vi "Write Content Bounds Width.vi"(8 "error in (no error)":errorcluster, 10 "ContentBounds.Width":u32, 11 "SceneGraphDisplay.lvclass in":refnum<class "SceneGraphDisplay.lvclass">) -> (0 "error out":errorcluster, 3 "SceneGraphDisplay.lvclass out":refnum<class "SceneGraphDisplay.lvclass">)   [LabVIEW 2015, in "SceneGraphDisplay.lvclass"]
uses:
  SceneGraphDisplay.lvclass
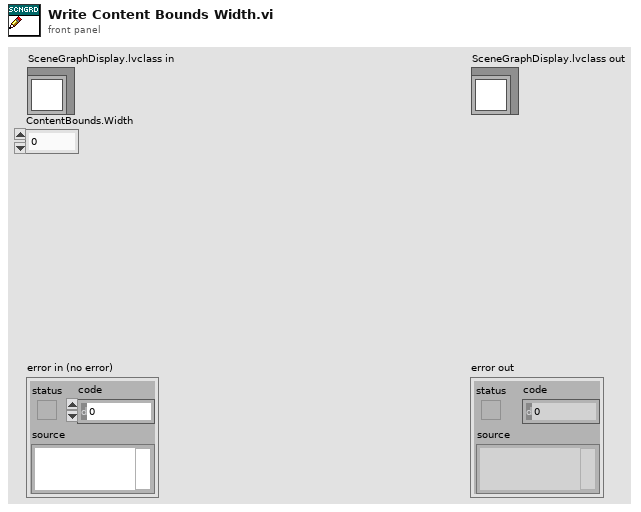
[diagram p1: front panel]
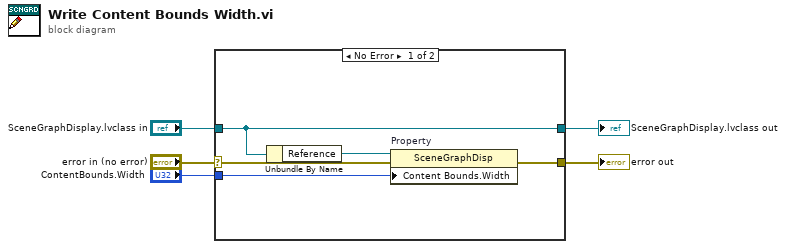
[diagram p0: block diagram]
diagram:
  n1 = case shown="No Error" "error in (no error)" {
    selector: "error in (no error)" -> [w6 w12]
    tunnel: [w10 w12] -> w4
    tunnel: [w8 w11] -> w2
    tunnel: "SceneGraphDisplay.lvclass in" -> [w8 w11]
    tunnel: "ContentBounds.Width" -> [w9 _]
    frame No Error {
      n2 = Unbundle By Name(w8) -> ("Reference"=w7:refnum<vi>)
      n3 = property on="Property" class="SceneGraphDisp"(reference=w7, error in=w6, "Content Bounds.Width"=w9) -> (error out=w10:errorcluster)  [unwired: 1 out]
    }
    frame Error {
    }
  }
  "error out" <- w4
  "SceneGraphDisplay.lvclass out" <- w2
